vi "Color Sensor V3 Get CIE XYZ.vi"(8 "error in (no error)":errorcluster, 11 "ColorSensorDevRef":T2={"I2CDevRef"={"DevStatus"={"status"=FALSE, "code"=0, "source"=""}, "Device Address"=0, "Handle"=0, "I2C Bus"=enum."Invalid"}} {"I2CDevRef"."Device Address" format="%.0x"}) -> (0 "error out":errorcluster, 2 "CIE XYZ":cluster{"X":dbl, "Y":dbl, "Z":dbl}, 3 "ColorSensorDevRef out":T2={"I2CDevRef"={"DevStatus"={"status"=FALSE, "code"=0, "source"=""}, "Device Address"=0, "Handle"=0, "I2C Bus"=enum."Invalid"}} {"I2CDevRef"."Device Address" format="%.0x"})   [LabVIEW 2019]
uses:
  TypeDef/Color Sensor V3 DevRef.ctl
  <vilib>/Rock Robotics/WPI/I2C/WPI_I2CDevRef.ctl
  <vilib>/Rock Robotics/SystemInterfaces/i2clib/i2c_bus.ctl
  <vilib>/Analysis/Matrix/Datatypes/RealMatrix.ctl
  <vilib>/Analysis/baseanly.llb/Real A x B.vi
  <vilib>/Analysis/Matrix/NI_Matrix.lvlib
  <vilib>/Analysis/NI_AALBase.lvlib
panel:
  out "A x B":T1
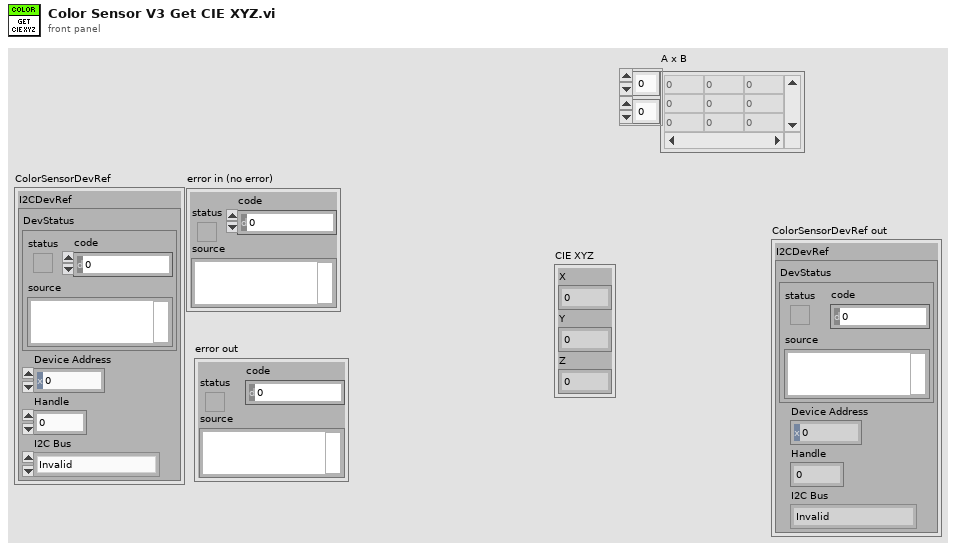
[diagram p1: front panel]
types:
  T1 = typedef "NI_Matrix.lvlib/RealMatrix.ctl" = dbl[][]
  T2 = typedef "Color Sensor V3 DevRef.ctl" = cluster{"I2CDevRef":T3}
  T3 = typedef "WPI_I2CDevRef.ctl" = cluster{"DevStatus":errorcluster, "Device Address":u8, "Handle":i32, "I2C Bus":T4}
  T4 = typedef "i2c_bus.ctl" = enum16{"I2C On-Board", "I2C MXP", "Invalid"}
  T5 = cluster{"Red":u32, "Green":u32, "Blue":u32, "IR":u32}
  T6 = cluster{"Real Matrix Element":dbl, "Real Matrix Element":dbl, "Real Matrix Element":dbl}
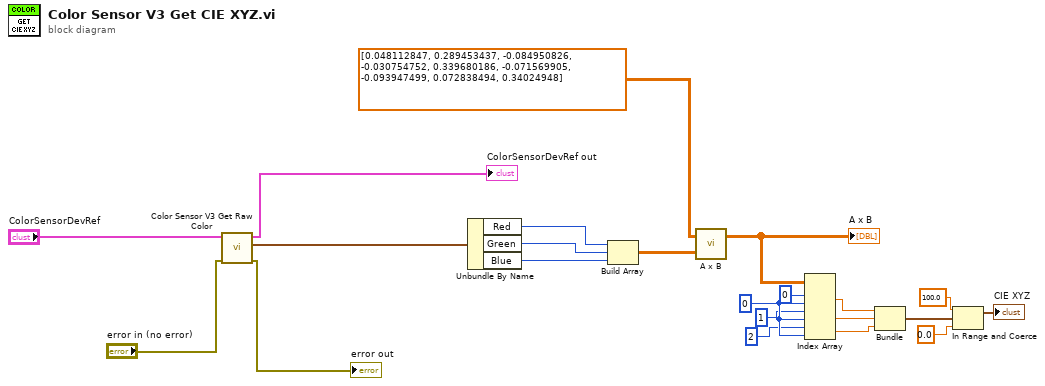
[diagram p0: block diagram]
diagram:
  w11 = 0 ("disabled index (col)")
  n1 = call "Color Sensor V3 Get Raw Color.vi"("error in (no error)"="error in (no error)", "ColorSensorDevRef"="ColorSensorDevRef") -> ("error out"=→"error out":errorcluster, "Raw Color"=w18:T5, "ColorSensorDevRef out"=→"ColorSensorDevRef out":T2)  [unwired: 7 in]
  n2 = Unbundle By Name(w18) -> ("Red"=w17:u32, "Green"=w16:u32, "Blue"=w15:u32)
  n3 = Build Array(w17, w16, w15) -> (w14:T1)
  n4 = call-poly <vilib>:"A x B.vi"("B"=w14, "A"=T1 [[0.048112847, 0.289453437, -0.084950826], [-0.030754752, 0.339680186, -0.071569905], [-0.093947499, 0.072838494, 0.34024948]] ("appended array")) -> ("A x B"=w12:T1)  [unwired: 1 out]
  "A x B" <- w12
  n5 = Index Array(array=w12, index (row) #1=0 ("disabled index (col)"), index (col) #1=w11, index (row) #2=1 ("disabled index (col)"), index (col) #2=w11, index (row) #3=2 ("disabled index (col)"), index (col) #3=w11) -> (element #1=w7:dbl, element #2=w6:dbl, element #3=w5:dbl)
  n6 = Bundle("Real Matrix Element"=w7, "Real Matrix Element"=w6, "Real Matrix Element"=w5) -> (w2:T6)  [unwired: 1 in]
  n7 = In Range and Coerce(upper limit=100.0 ("X"), x=w2, lower limit=0.0 ("X")) -> (coerced(x)=→"CIE XYZ":T6)  [unwired: 1 out]
